vi "DOPsetMeasuremen.vi"(2 "error in (no error)":errorcluster, 3 "CH":u8, 4 "VISA resource name":refnum<visa-resource-name>) -> (0 "error out":errorcluster, 1 "VISA resource name out":refnum<visa-resource-name>)   [LabVIEW 2018]
panel:
  # "设定测量\n测量1 脉宽\n测量2 频率"
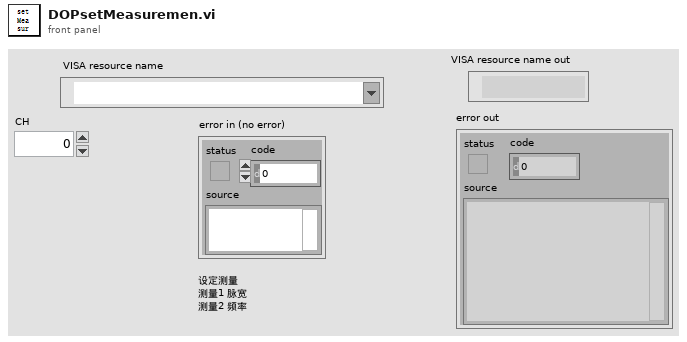
[diagram p1: front panel]
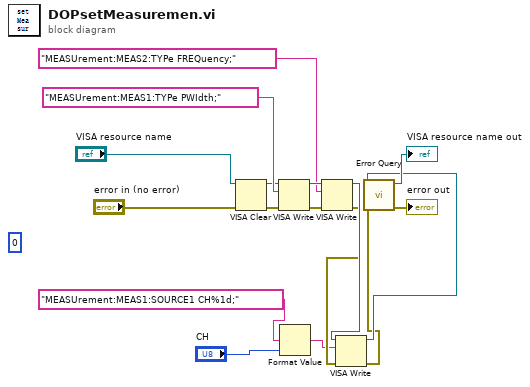
[diagram p0: block diagram]
diagram:
  (unwired) 0
  n1 = VISA Clear(VISA resource name="VISA resource name", error in (no error)="error in (no error)") -> (VISA resource name out=w13:refnum<visa-resource-name>, error out=w12:errorcluster)
  n2 = VISA Write(VISA resource name=w13, write buffer="MEASUrement:MEAS1:TYPe PWIdth;", error in (no error)=w12) -> (VISA resource name out=w16:refnum<visa-resource-name>, error out=w14:errorcluster)  [unwired: 1 out]
  n3 = Format Value(format string="MEASUrement:MEAS1:SOURCE1 CH%1d;", value (0)="CH") -> (output string=w1:string)  [unwired: 1 in]
  n4 = VISA Write(VISA resource name=w16, write buffer="MEASUrement:MEAS2:TYPe FREQuency;", error in (no error)=w14) -> (VISA resource name out=w5:refnum<visa-resource-name>, error out=w4:errorcluster)  [unwired: 1 out]
  n5 = VISA Write(VISA resource name=w5, write buffer=w1, error in (no error)=w4) -> (VISA resource name out=w3:refnum<visa-resource-name>, error out=w2:errorcluster)  [unwired: 1 out]
  n6 = call "Error Query.vi"("error in (no error)"=w2, "VISA resource name"=w3) -> ("error out"=→"error out":errorcluster, "VISA resource name out"=→"VISA resource name out":refnum<visa-resource-name>)  [unwired: 6 in, 2 out]
